vi "Read DXF Circle.vi"(8 "error in (no error)":errorcluster, 11 "path":path=path "D:/Git/Graph-Extensions-LabVIEW-master/LV2014/dxf/163_CAD2000_.dxf") -> (0 "error out":errorcluster, 2 "Radius":dbl[](array[numeric]), 3 "XY graph":cluster{dbl[], dbl[]}[](array[cluster]), 4 "Y":dbl[](array[numeric]), 5 "X":dbl[](array[numeric]))   [LabVIEW 2020, in "Graph Module.lvlib"]
uses:
  Graph Module.lvlib
  C:/Users/Fred Guo/Desktop/GarphView/Graph-Extensions-LabVIEW-master/Libraries/Graph Module/netDxf_2.4.2/bin/Release/netDxf.dll
  netDxf_2.4.2/bin/Release/netDxf.dll
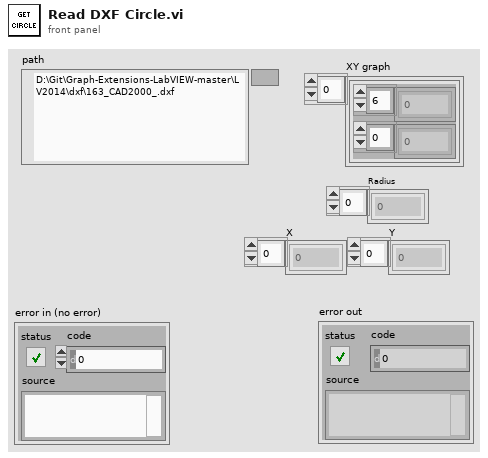
[diagram p1: front panel]
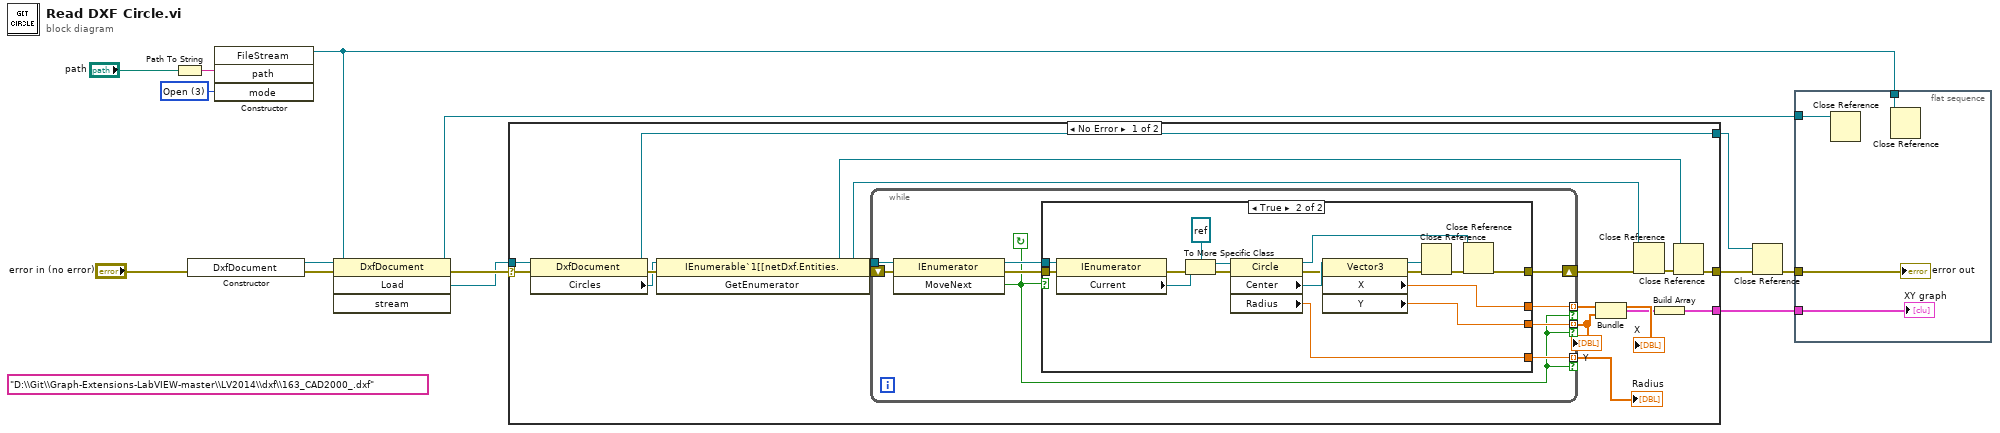
[diagram p0: block diagram]
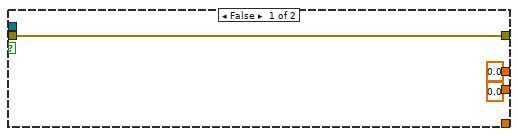
[diagram p2: hidden frame]
diagram:
  w4 = 3 items=["CreateNew"=1, "Create"=2, "Open"=3, "OpenOrCreate"=4, "Truncate"=5, "Append"=6] ("mode")
  (unwired) "D:\\Git\\Graph-Extensions-LabVIEW-master\\LV2014\\dxf\\163_CAD2000_.dxf" ("string")
  n1 = Path To String(path="path") -> (string=w3:string)
  n2 = constructor class="DxfDocument"(error in="error in (no error)") -> (reference out=w2:refnum<k24>, error out=w8:errorcluster)  [unwired: 2 in, 1 out]
  n3 = constructor class="FileStream"("path"=w3, "mode"=w4) -> (reference out=w1:refnum<k24>)  [unwired: 3 in, 4 out]
  n4 = invoke class="DxfDocument" method="Load"(reference=w2, error in=w8, "stream"=w1) -> (reference out=w5:refnum<k24>, error out=w7:errorcluster, "Load"=w6:refnum<k24>)  [unwired: 1 in, 1 out]
  n5 = case shown="No Error" w7 {
    selector: w7 -> [w23 w61]
    tunnel: w6 -> [w17 w60]
    tunnel: [w18 w60] -> w14
    tunnel: [w24 w61] -> w13
    tunnel: [w19 _] -> w12
    frame No Error {
      n6 = property class="DxfDocument"(reference=w17, error in=w23) -> (reference out=w18:refnum<k24>, error out=w29:errorcluster, "Circles"=w16:refnum<k24>)
      n7 = invoke class="IEnumerable`1[[netDxf.Entities." method="GetEnumerator"(reference=w16, error in=w29) -> (reference out=w25:refnum<k24>, error out=w30:errorcluster, "GetEnumerator"=w28:refnum<k24>)  [unwired: 1 in]
      n8 = while {
        tunnel: [w34] -> w22 mode=indexing if=w31
        tunnel: w28 -> [w36]
        shift-right: [w39] -> w27
        shift-left: w30 -> [w35]
        tunnel: [w33] -> w21 mode=indexing if=w31
        tunnel: [w32] -> w15 mode=indexing if=w31
        stop <- w31 continue-if-true
        n9 = invoke class="IEnumerator" method="MoveNext"(reference=w36, error in=w35) -> (reference out=w38:refnum<k24>, error out=w37:errorcluster, "MoveNext"=w31:bool)  [unwired: 1 in]
        n10 = case shown="True" w31 {
          tunnel: [w42 w59] -> w39
          tunnel: w38 -> [_ w47]
          tunnel: w37 -> [w42 w46]
          tunnel: [0.0 ("X") w45] -> w34
          tunnel: [0.0 ("Y") w44] -> w33
          tunnel: [_ w43] -> w32
          frame False {
          }
          frame True {
            n11 = property class="IEnumerator"(reference=w47, error in=w46) -> (error out=w48:errorcluster, "Current"=w49:refnum<k24>)  [unwired: 1 out]
            n12 = To More Specific Class(target class=refnum<k24> refnum ("new reference"), reference=w49, error in=w48) -> (specific class reference=w57:refnum<k24>, error out=w54:errorcluster)
            n13 = property class="Circle"(reference=w57, error in=w54) -> (reference out=w51:refnum<k24>, error out=w55:errorcluster, "Center"=w56:refnum<k24>, "Radius"=w43:dbl)
            n14 = property class="Vector3"(reference=w56, error in=w55) -> (reference out=w53:refnum<k24>, error out=w52:errorcluster, "X"=w45:dbl, "Y"=w44:dbl)
            n15 = Close Reference(reference=w53, error in (no error)=w52) -> (error out=w50:errorcluster)
            n16 = Close Reference(reference=w51, error in (no error)=w50) -> (error out=w59:errorcluster)
          }
        }
      }
      "Radius" <- w15
      "X" <- w22
      "Y" <- w21
      n17 = Bundle(w22, w21) -> (w20:cluster{dbl[], dbl[]})  [unwired: 1 in]
      n18 = Close Reference(reference=w28, error in (no error)=w27) -> (error out=w26:errorcluster)
      n19 = Build Array(w20) -> (w19:cluster{dbl[], dbl[]}[])
      n20 = Close Reference(reference=w25, error in (no error)=w26) -> (error out=w24:errorcluster)
    }
    frame Error {
    }
  }
  n21 = Close Reference(reference=w14, error in (no error)=w13) -> (error out=w10:errorcluster)
  n22 = flat-sequence {
    tunnel: w12 -> [w65]
    tunnel: w5 -> [w64]
    tunnel: w10 -> [w63]
    tunnel: w1 -> [w62]
    frame #0 {
      n23 = Close Reference(reference=w64) -> ()  [unwired: 1 in, 1 out]
      n24 = Close Reference(reference=w62) -> ()  [unwired: 1 in, 1 out]
      "error out" <- w63
      "XY graph" <- w65
    }
  }
